vi "Setup XNode Linker Reference.vi"(4 "VI to Monitor (owner)":path, 5 "error in":errorcluster, 6 "linkerClass (VI Sig)":T1(ring)=enum."VI Signature", 7 "Unique ID":string="_ANY UNIQUE NAME_", 8 "XRef":T2) -> (0 "error out":errorcluster)   [LabVIEW 2025, in "XNode Support.lvlib"]
uses:
  XNode Support.lvlib
  <vilib>/XNodeSupport/XNodeXNodeRef.ctl
  <vilib>/XNodeSupport/NI_XNodeSupport.lvlib
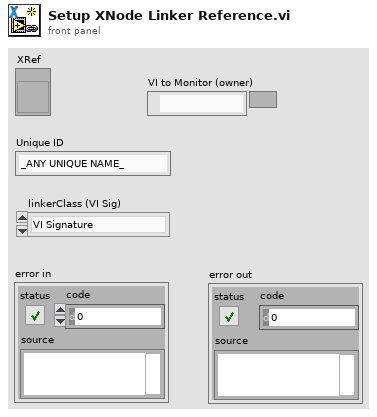
[diagram p1: front panel]
types:
  T1 = enum32{"Invalid Class", "File Path", "Variable", "Elemental IO", "VI Connector Pane", "VI Signature", "File No Warn", "Function Block Item", "Library Data"}
  T2 = typedef "NI_XNodeSupport.lvlib/XNodeXNodeRef.ctl" = refnum<vi>
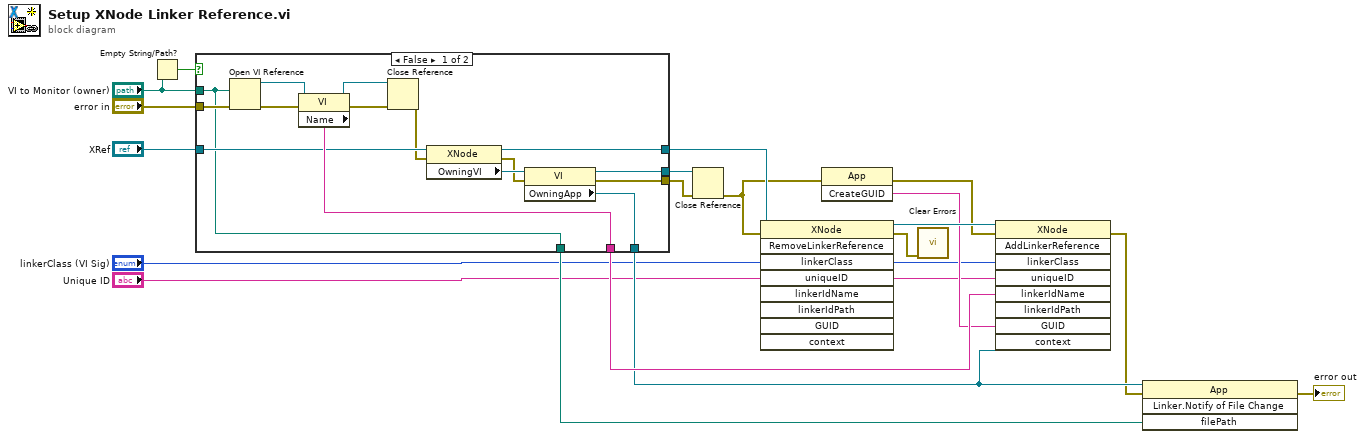
[diagram p0: block diagram]
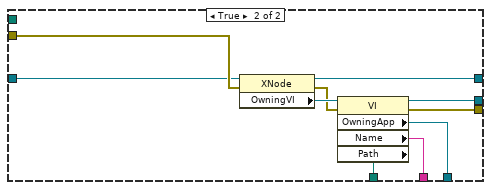
[diagram p2: hidden frame]
diagram:
  n1 = Empty String/Path?(string/path="VI to Monitor (owner)") -> (empty?=w5:bool)
  n2 = case shown="False" w5 {
    tunnel: [w34 w36] -> w19
    tunnel: [w22 w44] -> w18
    tunnel: [w33 w43] -> w16
    tunnel: [w32 w42] -> w2
    tunnel: [w31 w41] -> w4
    tunnel: "error in" -> [w30 w40]
    tunnel: "XRef" -> [w29 w39]
    tunnel: "VI to Monitor (owner)" -> [w22 _]
    tunnel: [w20 w35] -> w3
    frame False {
      n3 = Open VI Reference(vi path=w22, error in (no error)=w30) -> (vi reference=w27:refnum<vi>, error out=w26:errorcluster)  [unwired: 4 in]
      n4 = property class="VI"(reference=w27, error in=w26) -> (reference out=w21:refnum<vi>, error out=w25:errorcluster, "Name"=w34:string)
      n5 = Close Reference(reference=w21, error in (no error)=w25) -> (error out=w24:errorcluster)
      n6 = property class="XNode"(reference=w29, error in=w24) -> (reference out=w31:T2, error out=w23:errorcluster, "OwningVI"=w28:refnum<vi>)
      n7 = property class="VI"(reference=w28, error in=w23) -> (reference out=w20:refnum<vi>, error out=w32:errorcluster, "OwningApp"=w33:refnum<vi>)
    }
    frame True {
      n8 = property class="XNode"(reference=w39, error in=w40) -> (reference out=w41:T2, error out=w37:errorcluster, "OwningVI"=w38:refnum<vi>)
      n9 = property class="VI"(reference=w38, error in=w37) -> (reference out=w35:refnum<vi>, error out=w42:errorcluster, "OwningApp"=w43:refnum<vi>, "Name"=w36:string, "Path"=w44:path)
    }
  }
  n10 = Close Reference(reference=w3, error in (no error)=w2) -> (error out=w1:errorcluster)
  n11 = invoke class="XNode" method="RemoveLinkerReference"(reference=w4, error in=w1, "linkerClass"="linkerClass (VI Sig)", "uniqueID"="Unique ID") -> (reference out=w15:T2, error out=w11:errorcluster)  [unwired: 5 in, 7 out]
  n12 = invoke class="App" method="CreateGUID"(error in=w1) -> (error out=w12:errorcluster, "CreateGUID"=w13:string)  [unwired: 2 in, 1 out]
  n13 = call <vilib>:"Clear Errors.vi"("error in (no error)"=w11) -> ()  [unwired: 5 in, 2 out]
  n14 = invoke class="XNode" method="AddLinkerReference"(reference=w15, error in=w12, "linkerClass"="linkerClass (VI Sig)", "uniqueID"="Unique ID", "linkerIdName"=w19, "GUID"=w13, "context"=w16) -> (error out=w14:errorcluster)  [unwired: 2 in, 8 out]
  n15 = invoke class="App" method="Linker.Notify of File Change"(reference=w16, error in=w14, "filePath"=w18) -> (error out=→"error out":errorcluster)  [unwired: 1 in, 3 out]
